vi "Magnify.vi"(11 "Camera 2":T1(plugin-control)) -> ()   [LabVIEW 2012]
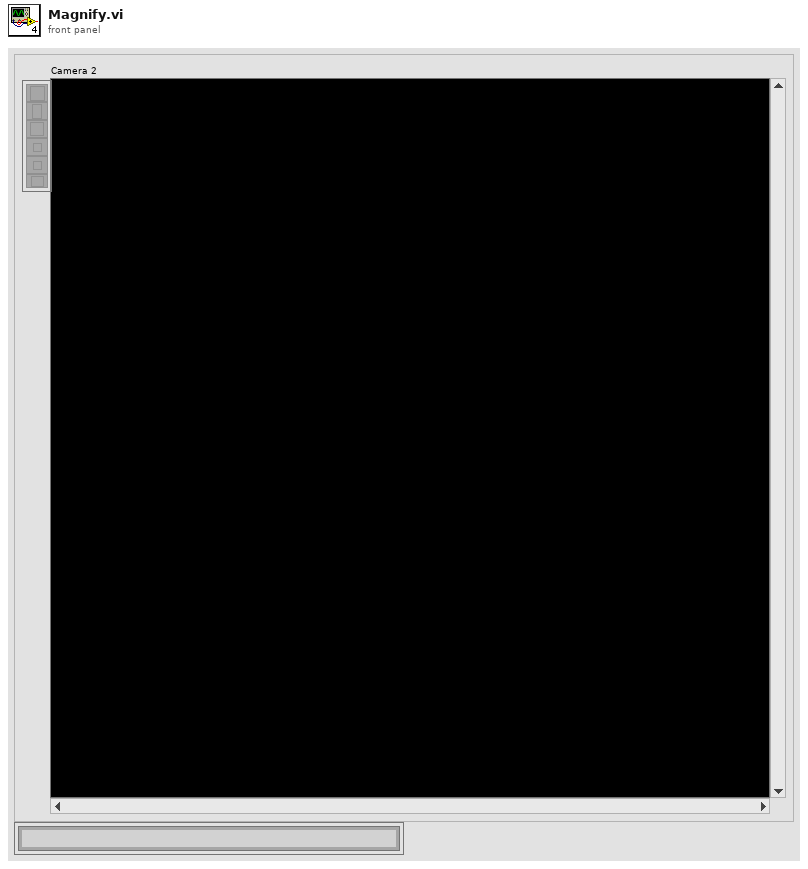
[diagram p1: front panel]
types:
  T1 = typedef "IMAQ Image.ctl" = refnum<image>
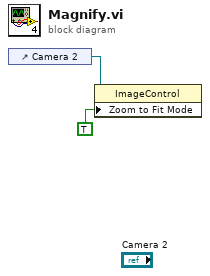
[diagram p0: block diagram]
diagram:
  n1 = control-ref of="Camera 2"() -> (w2:refnum<vi>)
  n2 = property on="Property Node" class="ImageControl"(reference=w2, "Zoom to Fit Mode"=TRUE) -> ()  [unwired: 1 in, 2 out]
